vi "仁莫密封检测系统.vi"() -> ()   [LabVIEW 2020]
uses:
  <vilib>/event_ctls.llb/eventvkey.ctl
  <vilib>/NI/Modbus Library/API/Master/Modbus Master.lvclass
  <vilib>/Utility/file.llb/Read Delimited Spreadsheet (string).vi
  <vilib>/NI/Modbus Library/Transmission Data Unit/RTU/RTU Data Unit.lvclass
  <vilib>/NI/Modbus Library/Master Function Definition/Master Function Definition.lvclass
  <vilib>/NI/Modbus Library/Network Protocol/Network Master/Serial/Serial Master.lvclass
panel:
  in  "sn":string
  out "MES状态":bool
  out "通讯状态":bool
  out "泄漏流量":string
  out "参数组别":string
  out "测试时间":string
  out "实时压力":string
  out "泄露压力":string
  out "门限压力":string
  out "目标压力":string
  out "测试 NG":string
  out "测试 OK":string
  out "测试结果":string
  out "测试总量":string
  out "实时压力(图)":dbl(graph)
  out "消息框+":string
  in  "清除计数":bool
  in  "设备启动":bool
  out "运行状态":string
  in  "设备停止":bool
  in  "阻断通讯":bool=TRUE
  out "运行状态":string
  out "失败原因":string
  in  "Exit":bool
  # "仁 莫 密 封 检 测 系 统"
  # "smcc"
  # "S"
  # "Pa"
  # "Pa"
  # "Pa"
  # "Pa"
  # "pcs"
  # "pcs"
  # "pcs"
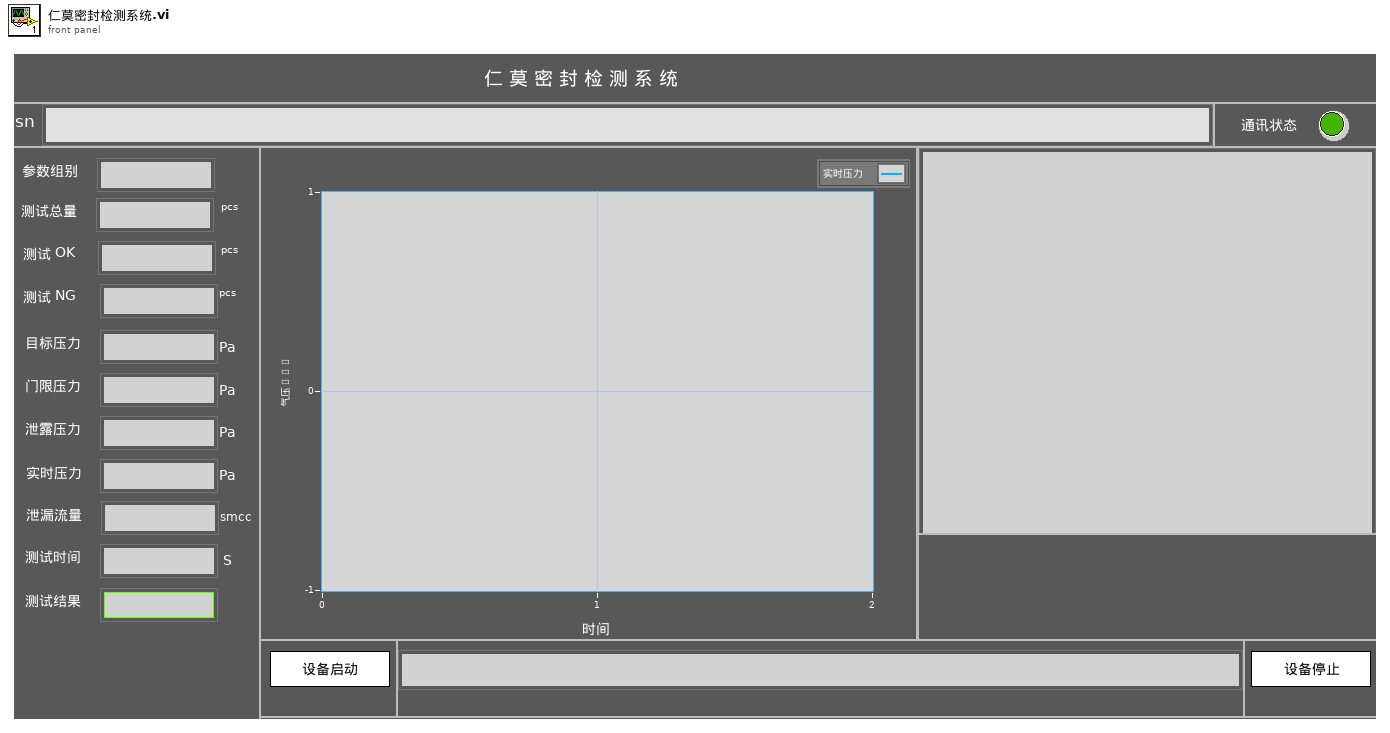
[diagram p1: front panel]
types:
  T1 = typedef "eventvkey.ctl" = enum16{"ASCII", "Enter", "Return", "Shift", "Ctrl", "Alt", "Cmd", "Opt", "Caps", "NumLock", "Clear", "Break", "Up", "Down", "Left", "Right", "Insert", "Delete", "Home", "End", "PageUp", "PageDown", "Escape", "Help", "Pause", "ScrollLock", "F1", "F2", "F3", "F4", "F5", "F6", "F7", "F8", "F9", "F10", "F11", "F12", "F13", "F14", "F15", "F16", "F17", "F18", "F19", "F20", "F21", "F22", "F23", "F24", "Play", "VolumeUp", "VolumeDown", "Mute", "Two Byte Char"}
  T2 = cluster{"地址":u16, "数量":u16, "寄存器值":u16[], "产品总数":string}[]
  T3 = enum32{"Invalid", "Standard", "Closed", "Hidden", "Minimized", "Maximized"}
  T4 = enum32{"invalid app kind", "Development System", "Run Time System", "Student Edition", "Embedded LabVIEW", "Evaluation", "Custom"}
  T5 = cluster{"地址":u16, "数量":u16, "寄存器值":u16[], "名称":string}[]
  T6 = cluster{"读取信息簇":cluster{"地址":u16, "数量":u16, "寄存器值":u16[], "名称":string}, "值解析":string}[]
  T7 = cluster{"温度instance":refnum<class "Modbus Master.lvclass">, "Core":cluster{"Current VI Reference":refnum<vi>, "Close Panel on Exit?":bool}, "serial master instance":refnum<class "Modbus Master.lvclass">, "进站OK":bool, "连接成功":bool, "正在运行":bool, "用户登录":bool, "A读保持寄存器信息组":cluster{"地址":u16, "数量":u16, "寄存器值":u16[], "名称":string}[], "A写入线圈信息组":cluster{"地址":u16, "布尔":bool, "名称":string}[], "A读多组线圈信息组":cluster{"地址":u16, "数量":u16, "名称":string, "线圈组":bool[]}[]}
  T8 = cluster{"连接成功":bool, "MB_实体":refnum<class "Modbus Master.lvclass">}
  T9 = cluster{"地址":u16, "数量":u16, "名称":string, "线圈组":bool[]}[]
  T10 = cluster{"Current VI Reference":refnum<vi>, "Close Panel on Exit?":bool}
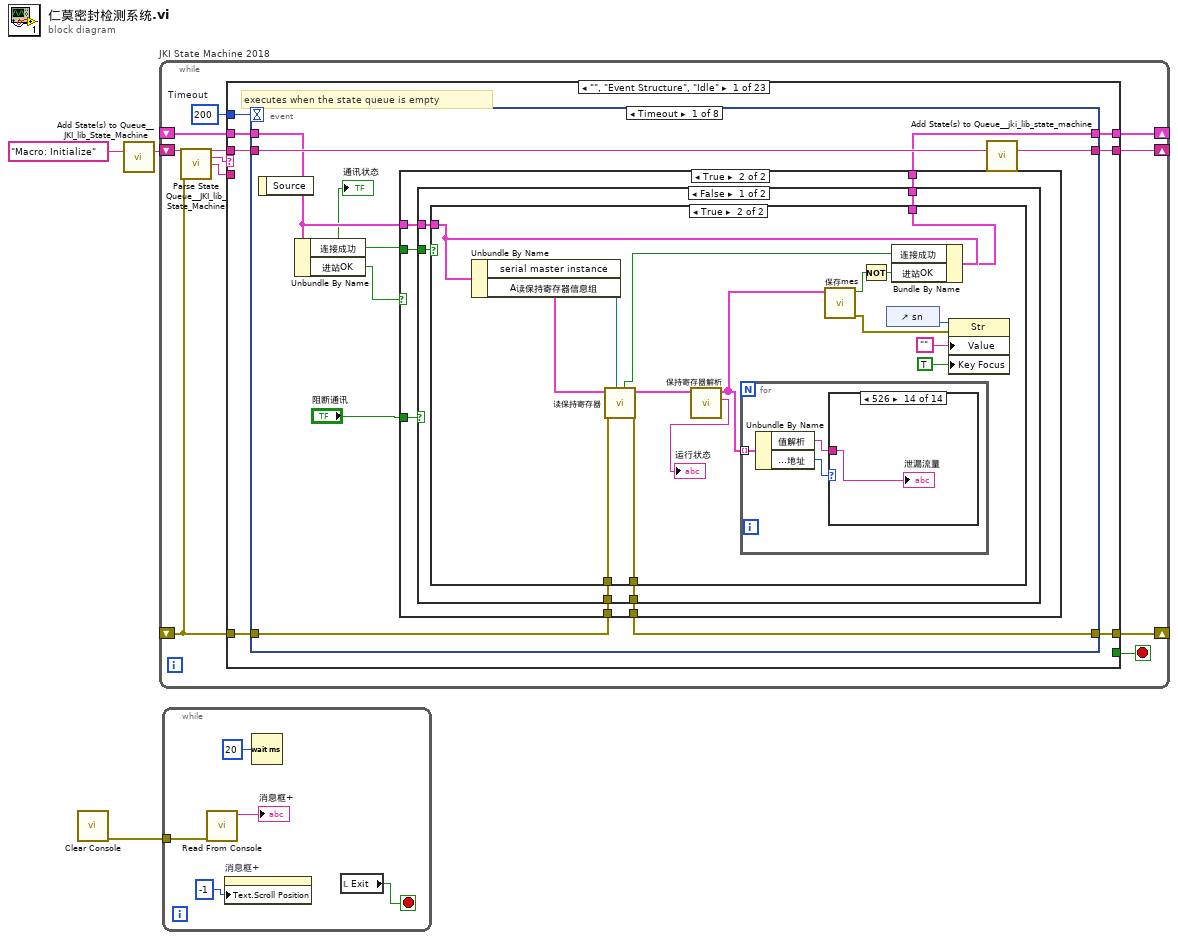
[diagram p0: block diagram]
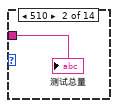
[diagram p5: hidden frame]
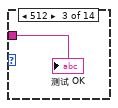
[diagram p6: hidden frame]
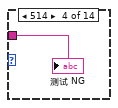
[diagram p7: hidden frame]
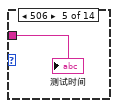
[diagram p8: hidden frame]
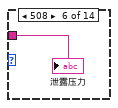
[diagram p9: hidden frame]
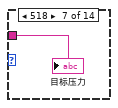
[diagram p10: hidden frame]
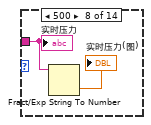
[diagram p11: hidden frame]
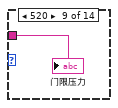
[diagram p12: hidden frame]
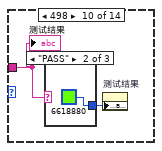
[diagram p13: hidden frame]
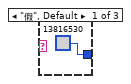
[diagram p14: hidden frame]
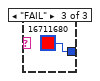
[diagram p15: hidden frame]
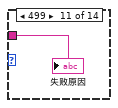
[diagram p16: hidden frame]
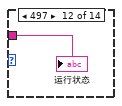
[diagram p17: hidden frame]
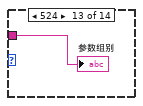
[diagram p18: hidden frame]
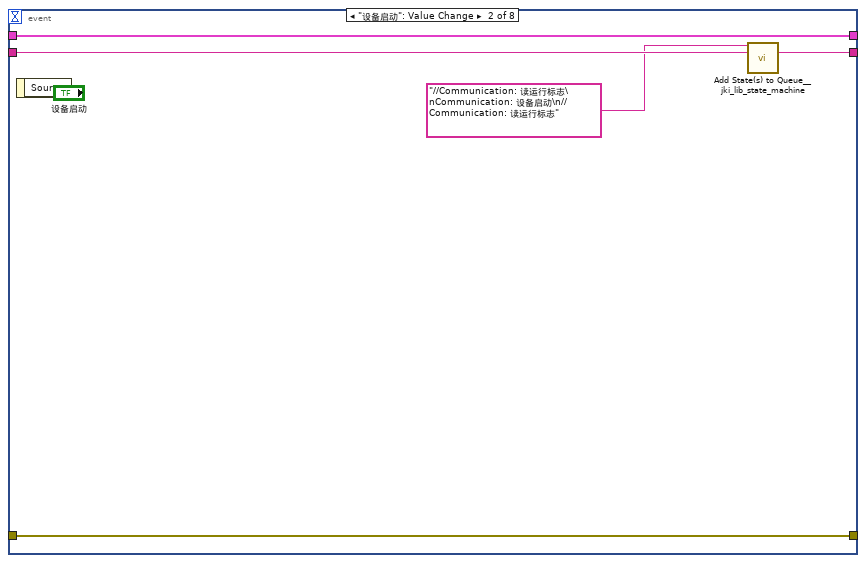
[diagram p20: hidden frame]
diagram:
  n1 = call "Clear Console.vi"() -> ("error out"=w1:errorcluster)  [unwired: 11 in]
  n2 = call <vilib>:"Add State(s) to Queue__JKI_lib_State_Machine.vi"("State(s) in (\"\")"="Macro: Initialize") -> ("States Out"=w3:string)  [unwired: 14 in]
  n3 = while "JKI State Machine 2018" {
    shift-right: [w7] -> _
    shift-left: _ -> [w6]
    shift-right: [w10] -> _
    shift-left: _ -> [w4]
    shift-right: [w9] -> _
    shift-left: w3 -> [w11]
    stop <- w8 stop-if-true
    w5 = 200  # Timeout
    n4 = call <vilib>:"Parse State Queue__JKI_lib_State_Machine.vi"("State Queue"=w11, "Error In (no error)"=w4) -> ("Remaining States"=w13:string, "Current State"=w14:string, "Arguments"=w12:string)  [unwired: 11 in]
    n5 = case shown="\"\", \"Event Structure\", \"Idle\"" w14 {
      selector: w14 -> [_ _ w190 _ _ _ _ _ _ _ _ _ _ _ _ _ _ _ _ _ _ _ _]
      tunnel: w13 -> [w21 w189 w194 w213 w220 w225 w229 w250 w259 w263 w277 w283 w294 w363 w368 w378 w382 w394 w406 w453 w485 w497 w502]
      tunnel: w12 -> [_ _ _ _ _ _ _ _ _ _ _ w278 w288 _ _ _ _ _ _ _ _ _ _]
      tunnel: w6 -> [w19 w186 w192 w206 w217 w223 w226 _ w255 w260 w275 w281 w290 w360 w365 w375 w379 w388 w400 w447 w478 w494 w499]
      tunnel: [w18 w187 w196 w210 errorcluster {"status"=FALSE, "code"=0, "source"=""} ("error out") w222 w227 w247 w256 w261 w274 w279 w291 w361 w366 w376 w380 w383 w403 w450 w482 w495 w500] -> w10
      tunnel: w4 -> [w17 w187 w195 w210 w215 w222 w227 w247 w253 w261 w274 w280 w292 w361 w366 w376 w380 w391 w404 w451 w483 w495 w500]
      tunnel: [w20 w188 w193 w212 w219 w224 w228 w249 w258 w262 w276 w282 w293 w362 w367 w377 w381 w393 w405 w452 w484 w496 w501] -> w9
      tunnel: [_ _ _ _ _ w221 _ _ _ _ _ _ _ _ _ _ _ _ _ _ _ _ _] -> w8
      tunnel: [w16 w186 w192 w211 w217 w223 w226 w248 w255 w260 w275 w281 w290 w360 w365 w375 w379 w386 w398 w445 w479 w494 w498] -> w7
      tunnel: w5 -> [w15 _ _ _ _ _ _ _ _ _ _ _ _ _ _ _ _ _ _ _ _ _ _]
      frame "", "Event Structure", "Idle" {
        # "executes when the state queue is empty"
        n6 = event shown="[0] Timeout" {
          selector: _ -> [_ _ _ _ _ _ _ _]
          dyn-events: _ -> [_ _ _ _ _ _ _ _]
          timeout: w15 -> [_ _ _ _ _ _ _ _]
          tunnel: w21 -> [w30 w89 w94 w100 w155 w169 w179 w185]
          tunnel: [w29 w88 w93 w99 w154 w168 w178 w184] -> w20
          tunnel: w19 -> [w28 w86 w91 w96 w152 w164 w176 w182]
          tunnel: [w26 w87 w92 w98 w153 w161 w177 w183] -> w18
          tunnel: w17 -> [w27 w87 w92 w98 w153 w162 w177 w183]
          tunnel: [w25 w86 w91 w95 w151 w163 w176 w182] -> w16
          event Timeout {
            n7 = event-data() -> ()  [unwired: 1 in, 1 out]
            n8 = Unbundle By Name(w28) -> ("连接成功"=w23:bool, "进站OK"=w22:bool)
            "通讯状态" <- w23
            n9 = case shown="True" w22 {
              tunnel: w28 -> [w32 w38]
              tunnel: w27 -> [w31 w37]
              tunnel: [w31 w36] -> w26
              tunnel: [w32 w35] -> w25
              tunnel: "阻断通讯" -> [_ w34]
              tunnel: w23 -> [_ w33]
              frame False {
              }
              frame True {
                n10 = case shown="False" w34 {
                  tunnel: w33 -> [w43 _]
                  tunnel: w38 -> [w42 w83]
                  tunnel: w37 -> [w41 w84]
                  tunnel: [w40 w84] -> w36
                  tunnel: [w39 w83] -> w35
                  frame False {
                    n11 = case shown="True" w43 {
                      tunnel: w42 -> [w44 w59]
                      tunnel: w41 -> [w45 w61]
                      tunnel: [w45 w60] -> w40
                      tunnel: [w44 w54] -> w39
                      frame False {
                      }
                      frame True {
                        n12 = Unbundle By Name(w59) -> ("serial master instance"=w58:refnum<class "Modbus Master.lvclass">, "A读保持寄存器信息组"=w57:T5)
                        n13 = call "读保持寄存器.vi"("MB_实体"=w58, "error in"=w61, "读保持寄存器信息组__输入"=w57) -> ("输出簇"=w60:errorcluster, "读保持寄存器信息组_输出"=w55:T5, "连接成功"=w56:bool)  [unwired: 6 in]
                        n14 = call "保持寄存器解析.vi"("A读保持寄存器信息组"=w55) -> ("运行状态"=→"运行状态":string, "参数值"=w53:T6)  [unwired: 9 in]
                        n15 = for {
                          tunnel: w53 -> [w63] mode=indexing
                          n16 = Unbundle By Name(w63) -> ("值解析"=w62:string, "读取信息簇.地址"=w64:u16)
                          n17 = case shown="526" w64 {
                            tunnel: w62 -> [_ w65 w66 w67 w68 w69 w70 w72 w73 w75 w79 w80 w81 w82]
                            frame Default {
                            }
                            frame 510 {
                              "测试总量" <- w65
                            }
                            frame 512 {
                              "测试 OK" <- w66
                            }
                            frame 514 {
                              "测试 NG" <- w67
                            }
                            frame 506 {
                              "测试时间" <- w68
                            }
                            frame 508 {
                              "泄露压力" <- w69
                            }
                            frame 518 {
                              "目标压力" <- w70
                            }
                            frame 500 {
                              n18 = Fract/Exp String To Number(string=w72) -> (number=→"实时压力(图)":dbl)  [unwired: 3 in, 1 out]
                              "实时压力" <- w72
                            }
                            frame 520 {
                              "门限压力" <- w73
                            }
                            frame 498 {
                              n19 = case shown="\"PASS\"" w75 {
                                tunnel: [u32 13816530 ("颜色盒") u32 6618880 u32 16711680] -> w74
                                frame "假", Default {
                                }
                                frame "PASS" {
                                }
                                frame "FAIL" {
                                }
                              }
                              n20 = property on="测试结果" class="Str"("Text.BGColor"=w74) -> ()  [unwired: 2 in, 2 out]
                              "测试结果" <- w75
                            }
                            frame 499 {
                              "失败原因" <- w79
                            }
                            frame 497 {
                              "运行状态" <- w80
                            }
                            frame 524 {
                              "参数组别" <- w81
                            }
                            frame 526 {
                              "泄漏流量" <- w82
                            }
                          }
                        }
                        n21 = call "保存mes.vi"("参数值"=w53) -> ("error out"=w48:errorcluster, "出站成功"=w51:bool)  [unwired: 9 in]
                        n22 = Not(x=w51) -> (.not. x?=w50:bool)
                        n23 = control-ref of="sn"() -> (w49:refnum<vi>)
                        n24 = Bundle By Name(cluster=w59, "连接成功"=w56, "进站OK"=w50) -> (w54:T7)
                        n25 = property on="属性节点" class="Str"(reference=w49, error in=w48, "Value"="", "Key Focus"=TRUE ("键选中")) -> ()  [unwired: 2 out]
                      }
                    }
                  }
                  frame True {
                  }
                }
              }
            }
            n26 = call <vilib>:"Add State(s) to Queue__jki_lib_state_machine.vi"("State(s) in (\"\")"=w30) -> ("States Out"=w29:string)  [unwired: 14 in]
          }
          event "设备启动": Value Change {
            n27 = event-data() -> ()  [unwired: 1 in, 1 out]
            n28 = call <vilib>:"Add State(s) to Queue__jki_lib_state_machine.vi"("State(s) in Front (\"\")"="//Communication: 读运行标志\nCommunication: 设备启动\n//Communication: 读运行标志", "State(s) in (\"\")"=w89) -> ("States Out"=w88:string)  [unwired: 13 in]
          }
          event "设备停止": Value Change {
            n29 = event-data() -> ()  [unwired: 1 in, 1 out]
            n30 = call <vilib>:"Add State(s) to Queue__jki_lib_state_machine.vi"("State(s) in Front (\"\")"="//Communication: 读运行标志\nCommunication: 设备停止\n//Communication: 读运行标志", "State(s) in (\"\")"=w94) -> ("States Out"=w93:string)  [unwired: 13 in]
          }
          event Menu Selection (User) {
            n31 = event-data() -> ("ItemTag"=w97:string)  [unwired: 1 in]
            n32 = case shown="\"历史数据路径配置\"" w97 {
              tunnel: w96 -> [w101 w102 w113 w124 w125 w127 w138]
              tunnel: [w101 w102 w113 w124 w125 w126 w137] -> w95
              frame "假", Default {
              }
              frame "历史数据查询" {
                n33 = stacked-sequence {
                  frame #0 {
                    n34 = call <vilib>:"Check if File or Folder Exists.vi"("path"=path "D:/MES" ("路径")) -> ("file or folder exists?"=w105:bool, "dup path"=w104:path)  [unwired: 8 in, 1 out]
                    n35 = case shown="False" w105 {
                      tunnel: w104 -> [w107 w108]
                      tunnel: [w106 w108] -> _
                      frame False {
                        n36 = Create Folder(path (use dialog)=w107) -> (created path=w106:path)  [unwired: 2 in, 2 out]
                      }
                      frame True {
                      }
                    }
                  }
                  frame #1 {
                    n37 = call <vilib>:"Space Constant.vi"() -> ("String"=w110:string)
                    n38 = Concatenate Strings("explorer" ("字符串"), w110, "D:\\MES" ("字符串")) -> (w112:string)
                    n39 = call <vilib>:"System Exec.vi"("command line"=w112) -> ()  [unwired: 7 in, 4 out]
                  }
                }
              }
              frame "MES日志查询" {
                n40 = stacked-sequence {
                  frame #0 {
                    n41 = call <vilib>:"Check if File or Folder Exists.vi"("path"=path "D:/Log" ("路径")) -> ("file or folder exists?"=w116:bool, "dup path"=w115:path)  [unwired: 8 in, 1 out]
                    n42 = case shown="False" w116 {
                      tunnel: w115 -> [w118 w119]
                      tunnel: [w117 w119] -> _
                      frame False {
                        n43 = Create Folder(path (use dialog)=w118) -> (created path=w117:path)  [unwired: 2 in, 2 out]
                      }
                      frame True {
                      }
                    }
                  }
                  frame #1 {
                    n44 = call <vilib>:"Space Constant.vi"() -> ("String"=w121:string)
                    n45 = Concatenate Strings("explorer" ("字符串"), w121, "D:\\Log" ("字符串")) -> (w123:string)
                    n46 = call <vilib>:"System Exec.vi"("command line"=w123) -> ()  [unwired: 7 in, 4 out]
                  }
                }
              }
              frame "IP配置" {
                n47 = call "IP配置.vi"() -> ()  [unwired: 11 in, 1 out]
              }
              frame "历史数据路径配置" {
                n48 = call "Path配置.vi"() -> ()  [unwired: 11 in, 1 out]
              }
              frame "通讯参数设置" {
                n49 = stacked-sequence {
                  tunnel: w127 -> [_ w132 _]
                  tunnel: [_ w129 _] -> w126
                  frame #0 {
                    n50 = local write "阻断通讯"(TRUE ("阻断通讯")) -> ()
                  }
                  frame #1 {
                    n51 = call "通讯参数设置.vi"() -> ("A设备簇"=w133:T8)  [unwired: 5 in]
                    n52 = Unbundle By Name(w133) -> ("MB_实体"=w131:refnum<class "Modbus Master.lvclass">, "连接成功"=w130:bool)
                    n53 = Bundle By Name(cluster=w132, "serial master instance"=w131, "连接成功"=w130) -> (w129:T7)
                  }
                  frame #2 {
                    n54 = local write "阻断通讯"(FALSE ("阻断通讯")) -> ()
                  }
                }
              }
              frame "本地控制" {
                n55 = call "本地控制.vi"() -> ("远程2"=w136:bool)  [unwired: 11 in]
                "MES状态" <- w136
                n56 = Not(x=w136) -> (.not. x?=w135:bool)
                n57 = Bundle By Name(cluster=w138, "用户登录"=w135, "进站OK"=w135) -> (w137:T7)
                n58 = global write "Global.vi" "产品进站"(w135) -> ()
                n59 = case shown="True" w136 {
                  frame False {
                    n60 = Current VI's Menubar() -> (w140:refnum<k9>)
                    n61 = Delete Menu Items(9:w140) -> (3:w139:refnum<k9>)  [unwired: 3 in, 1 out]
                    n62 = Insert Menu Items(7:string[] ["历史数据查询", "通讯参数设置", "MES配置", "MES日志查询", "本地控制", "温湿度设置"] ("L10n_item tags 1"), 9:w139) -> ()  [unwired: 4 in, 3 out]
                  }
                  frame True {
                    n63 = Current VI's Menubar() -> (w144:refnum<k9>)
                    n64 = Delete Menu Items(9:w144) -> (0:w142:errorcluster, 3:w143:refnum<k9>)  [unwired: 3 in]
                    n65 = Insert Menu Items(6:w142, 7:string[] ["用户登录", "历史数据查询", "通讯参数设置", "MES配置", "MES日志查询", "本地控制", "温湿度设置"] ("L10n_item tags 1"), 9:w143) -> ()  [unwired: 3 in, 3 out]
                  }
                }
              }
            }
            n66 = call <vilib>:"Add State(s) to Queue__jki_lib_state_machine.vi"("State(s) in (\"\")"=w100) -> ("States Out"=w99:string)  [unwired: 14 in]
          }
          event "sn": Key Down {
            n67 = event-data() -> ("VKey"=w150:T1)  [unwired: 1 in]
            n68 = Equal?(x=w150, y=eventvkey."Return" ("V键")) -> (x = y?=w148:bool)
            n69 = case shown="True" w148 {
              tunnel: [FALSE ("进站成功") TRUE ("进站成功")] -> w147
              frame False {
              }
              frame True {
                n70 = global write "Global.vi" "sn"("sn") -> ()
              }
            }
            n71 = global write "Global.vi" "产品进站"(w147) -> ()
            n72 = Bundle By Name(cluster=w152, "进站OK"=w147) -> (w151:T7)
            n73 = case shown="True" w147 {
              tunnel: ["" "Communication: 设备启动"] -> w146
              frame False {
              }
              frame True {
              }
            }
            n74 = call <vilib>:"Add State(s) to Queue__jki_lib_state_machine.vi"("State(s) in (\"\")"=w155, "State(s) at Back (\"\")"=w146) -> ("States Out"=w154:string)  [unwired: 13 in]
          }
          event "清除计数": Value Change {
            n75 = event-data() -> ()  [unwired: 1 in, 1 out]
            n76 = local write "清除计数"(FALSE) -> ()
            n77 = Unbundle By Name(w164) -> ("serial master instance"=w165:refnum<class "Modbus Master.lvclass">)
            n78 = disable-structure shown="禁用" {
              disable-tunnel: [w174 _] -> w166
              disable-tunnel: w165 -> [w173 _]
              disable-tunnel: w162 -> [w171 _]
              disable-tunnel: [w170 _] -> w161
              frame Disabled {
                n79 = call "写保持寄存器.vi"("MB_实体"=w173, "error in"=w171, "读保持寄存器信息组__输入"=T2 [{"地址"=510, "数量"=2, "寄存器值"=[0, 0], "产品总数"="产品总数"}, {"地址"=512, "数量"=2, "寄存器值"=[0, 0], "产品总数"="合格数量"}, {"地址"=514, "数量"=2, "寄存器值"=[0, 0], "产品总数"="泄露数量"}]) -> ("输出簇"=w170:errorcluster, "连接成功"=w174:bool)  [unwired: 7 in]
              }
              frame Enabled {
              }
            }
            n80 = Bundle By Name(cluster=w164, "连接成功"=w166) -> (w163:T7)
            n81 = call <vilib>:"Add State(s) to Queue__jki_lib_state_machine.vi"("State(s) in (\"\")"=w169) -> ("States Out"=w168:string)  [unwired: 14 in]
          }
          event "Exit": Value Change {
            # "Exit Button Value Change (pressed) Event\n(this executes Macro: Exit to terminate the VI)"
            n82 = event-data() -> ()  [unwired: 1 in, 1 out]
            n83 = call <vilib>:"Add State(s) to Queue__jki_lib_state_machine.vi"("State(s) in Front (\"\")"="Macro: Exit", "State(s) in (\"\")"=w179) -> ("States Out"=w178:string)  [unwired: 13 in]
          }
          event Panel Close? {
            # "Discard the event because we'll close the front panel ourselves in Macro: Exit"
            # "Close Panel button (pressed) Event\n(this executes Macro: Exit to terminate the VI)"
            n84 = event-data() -> ()  [unwired: 1 in, 1 out]
            n85 = call <vilib>:"Add State(s) to Queue__jki_lib_state_machine.vi"("State(s) in Front (\"\")"="Macro: Exit", "State(s) in (\"\")"=w185) -> ("States Out"=w184:string)  [unwired: 13 in]
            n86 = event-data("Discard?"=TRUE) -> ()  [unwired: 1 in, 1 out]
          }
        }
      }
      frame "---------- Core ----------" {
        # "Do not put any code in this frame.\n(it is a separator no-op)"
        n87 = call <vilib>:"Add State(s) to Queue__jki_lib_state_machine.vi"("State(s) in (\"\")"=w189) -> ("States Out"=w188:string)  [unwired: 14 in]
      }
      frame Default {
        w199 = 42 items=["No error", "Argument error", "Memory is full", "Out of zone", "End of file", "File already open", "Generic file I/O error", "File not found", "File permission error", "Disk is full", "Duplicate path", "Too many files open", "System feature not enabled", "Resource file not found", "Cannot add resource", "Resource not found", "Image not found", "Image memory error", "Pen does not exist", "Config type invalid", "Config token not found", "Config parse error", "Config memory error", "Bad external code format", "Bad external code offset", "External code not present", "Null window", "Destroy window error", "Null menu", "Print aborted", "Bad print record", "Print driver error", "Windows error during printing", "Memory error during printing", "Print dialog error", "Generic print error", "Invalid device refnum", "Device not found", "Device parameter error", "Device unit error", "Cannot open device", "Device call aborted", "Generic error", "Cancelled by user", "Object ID too low", "Object ID too high", "Object not in heap", "Unknown heap", "Unknown object (invalid DefProc)", "Unknown object (DefProc not in table)", "Message out of range", "Invalid (null) method", "Unknown message", "Manager call not supported", "Bad address", "Network operation in progress", "Network operation timed out", "Connection is busy", "Network attribute not supported", "Network error", "Address in use", "System out of memory", "Connection aborted", "Connection refused", "Not connected", "Already connected", "Connection closed", "Initialization error (interapplication manager)", "Bad occurrence", "Wait on unbound occurrence handler", "Occurrence queue overflow", "Datalog type conflict", "Unused", "Unrecognized type (interapplication manager)", "Memory corrupt", "Failed to make temporary DLL", "Old CIN version", "Drag socket not found", "Failed to load drop-object", "Failed to register OLE object", "Failed to release OLE object", "Format specifier type mismatch", "Unknown format specifier", "Too few format specifiers", "Too many format specifiers", "Scan failed", "Newer CIN version", "Error converting to variant", "Runtime menu error", "Password tampered", "Variant attribute not found", "Incompatible variant data type", "Event data is not available", "Event Store is not present", "Occurrence is not found", "Event Queue is not created", "Event info is not available", "Refnum passed is NULL", "Error retrieving Class GUID", "Error retrieving CoClass GUID", "Error retrieving TypeLib GUID.", "Bad built application magic bytes.", "Specific driver is different from the specific driver associated with the Logical Name.", "There is no session opened to the class driver.", "Max Error", "MAX - Error with config objects", "MAX - Error loading configuration", "MAX - Group not supported"]
        # "Current State"
        # "Do not delete, rename, or modify this frame.\n(this is used to capture unhandled states and typos)"
        # "Handle mistyped state name (developer tool)"
        n88 = Format Into String(format string="Software Exception: Unhandled State \"%s\"." ("message"), error in=w195, w190) -> (resulting string=w198:string, error out=w197:errorcluster)  [unwired: 1 in]
        n89 = call <vilib>:"Error Cluster From Error Code.vi"("show call chain? (False)"=TRUE, "error in (no error)"=w197, "error message (\"\")"=w198, "error code (0)"=w199) -> ("error out"=w196:errorcluster)  [unwired: 5 in]
        n90 = call <vilib>:"Add State(s) to Queue__jki_lib_state_machine.vi"("State(s) in (\"\")"=w194) -> ("States Out"=w193:string)  [unwired: 14 in]
      }
      frame "Initialize Core Data" {
        # "Do not delete, rename, or modify this frame.\n(this is used to determine panel behavior on exit)"
        # "originally closed?"
        # "exe?"
        # "If panel starts closed or is an EXE, then close it when we exit"
        n91 = property class="VI"() -> ("FP.State"=w203:T3)  [unwired: 2 in, 2 out]
        n92 = property class="App"() -> ("App.Kind"=w209:T4)  [unwired: 2 in, 2 out]
        n93 = control-ref of="Current VI Reference"() -> (w204:refnum<vi>)
        n94 = Equal?(x=w203, y=T3."Closed" ("Front Panel Window:State")) -> (x = y?=w201:bool)
        n95 = Equal?(x=w209, y=T4."Run Time System" ("Application:Kind")) -> (x = y?=w207:bool)
        n96 = Or(x=w201, y=w207) -> (x .or. y?=w205:bool)
        n97 = Bundle By Name(cluster=w206, "Core.Current VI Reference"=w204, "Core.Close Panel on Exit?"=w205) -> (w211:T7)
        n98 = call <vilib>:"Add State(s) to Queue__jki_lib_state_machine.vi"("State(s) in (\"\")"=w213) -> ("States Out"=w212:string)  [unwired: 14 in]
      }
      frame "Error Handler" {
        # "Handle any errors here.\nYou can also output any states to clean-up after errors occur"
        # "Clear error"
        n99 = Unbundle By Name(w215) -> ("source"=w214:string)
        n100 = One Button Dialog(message=w214) -> ()  [unwired: 1 in, 1 out]
        n101 = call <vilib>:"Add State(s) to Queue__jki_lib_state_machine.vi"("State(s) in Front (\"\")"="/* Post Error States", "State(s) in (\"\")"=w220) -> ("States Out"=w219:string)  [unwired: 13 in]
      }
      frame "Exit" {
        w221 = TRUE
        # "Do not put any code in this frame.\n(No errors that occur here will be handled.)"
        n102 = local write "Exit"(w221) -> ()
        n103 = call <vilib>:"Add State(s) to Queue__jki_lib_state_machine.vi"("State(s) in (\"\")"=w225) -> ("States Out"=w224:string)  [unwired: 14 in]
      }
      frame "---------- Data ----------" {
        # "Do not put any code in this frame.\n(It is a separator no-op. You can make a copy of this frame to create a new Data frame)"
        n104 = call <vilib>:"Add State(s) to Queue__jki_lib_state_machine.vi"("State(s) in (\"\")"=w229) -> ("States Out"=w228:string)  [unwired: 14 in]
      }
      frame "Data: Initialize" {
        w230 = refnum<class "Modbus Master.lvclass"> refnum  # 温度instance
        w231 = FALSE ("MES状态")
        w232 = FALSE  # 进站OK
        w239 = TRUE  # 用户登录
        w240 = FALSE  # 正在运行
        w241 = T5 [{"地址"=510, "数量"=2, "寄存器值"=[0, 0], "名称"="产品总数"}, {"地址"=512, "数量"=2, "寄存器值"=[0, 0], "名称"="合格数量"}, {"地址"=514, "数量"=2, "寄存器值"=[0, 0], "名称"="泄露数量"}, {"地址"=506, "数量"=2, "寄存器值"=[0, 0], "名称"="1测试时间"}, {"地址"=508, "数量"=2, "寄存器值"=[0, 0], "名称"="1测试泄漏"}, {"地址"=518, "数量"=2, "寄存器值"=[0, 0], "名称"="1#目标压力"}, {"地址"=498, "数量"=1, "寄存器值"=[0, 0], "名称"="1#测试结果"}, {"地址"=500, "数量"=2, "寄存器值"=[0, 0], "名称"="实时压力"}, {"地址"=520, "数量"=2, "寄存器值"=[], "名称"="门限压力"}, {"地址"=499, "数量"=1, "寄存器值"=[], "名称"="失败原因"}, {"地址"=497, "数量"=1, "寄存器值"=[], "名称"="运行状态"}, {"地址"=524, "数量"=2, "寄存器值"=[], "名称"="参数组别"}, {"地址"=526, "数量"=4, "寄存器值"=[], "名称"="泄漏流量"}]  # A读保持寄存器信息组
        w242 = T9 [{"地址"=507, "数量"=1, "名称"="1测试结束标志", "线圈组"=[FALSE, TRUE]}]  # A读多组线圈信息组
        w243 = cluster{"地址":u16, "布尔":bool, "名称":string}[] [{"地址"=50, "布尔"=FALSE, "名称"="启动"}, {"地址"=51, "布尔"=FALSE, "名称"="停止"}]  # A写入线圈信息组
        w244 = FALSE  # 连接成功
        w245 = refnum<class "Modbus Master.lvclass"> refnum  # serial master instance
        w246 = T10 {"Current VI Reference"=refnum, "Close Panel on Exit?"=FALSE}  # Core
        # "Initialize the shift-register data, here.\n(data names are defined by what you wire into the bundle function)"
        n105 = call <vilib>:"Application Directory.vi"() -> ("Application Directory"=w237:path)
        n106 = Build Path(base path=w237, name or relative path=path "data/mes.cfg") -> (appended path=w238:path)
        n107 = call-poly <vilib>:"Read Delimited Spreadsheet.vi"("file path (dialog if empty)"=w238, "delimiter (\\t)"="::" ("delimiter (\\t)")) -> ("all rows"=w233:string[][])  [unwired: 8 in, 5 out]
        n108 = call "mes初始化.vi"("mes"=w233) -> ()  [unwired: 11 in]
        n109 = disable-structure shown="禁用" {
          frame Disabled {
            n110 = global write "Global.vi" "MES状态"(TRUE ("MES状态")) -> ()
          }
          frame Enabled {
          }
        }
        n111 = global write "Global.vi" "正在运行"(w231) -> ()
        n112 = global write "Global.vi" "产品进站"(w231) -> ()
        n113 = global write "Global.vi" "运行状态时间点"(dbl[] [0.0, 0.0, 0.0, 0.0, 0.0, 0.0, 0.0, 0.0, 0.0] ("运行状态时间点")) -> ()
        n114 = Bundle("温度instance"=w230, "Core"=w246, "serial master instance"=w245, "进站OK"=w232, "连接成功"=w244, "正在运行"=w240, "用户登录"=w239, "A读保持寄存器信息组"=w241, "A写入线圈信息组"=w243, "A读多组线圈信息组"=w242) -> (w248:T7)  [unwired: 1 in]
        n115 = call <vilib>:"Add State(s) to Queue__jki_lib_state_machine.vi"("State(s) in (\"\")"=w250) -> ("States Out"=w249:string)  [unwired: 14 in]
      }
      frame "Data: Cleanup" {
        # "Cleanup any data and references, here.\n(this is called automatically, by the Macro: Exit)"
        n116 = Unbundle By Name(w255) -> ("Core.Current VI Reference"=w257:refnum<vi>, "serial master instance"=w254:refnum<class "Modbus Master.lvclass">)
        n117 = call-dynamic "Shutdown.vi"("error in"=w253, "Modbus master in"=w254) -> ("error out"=w252:errorcluster)  [unwired: 9 in]
        n118 = Close Reference(reference=w257, error in (no error)=w252) -> (error out=w256:errorcluster)
        n119 = call <vilib>:"Add State(s) to Queue__jki_lib_state_machine.vi"("State(s) in (\"\")"=w259) -> ("States Out"=w258:string)  [unwired: 14 in]
      }
      frame "---------- UI ----------" {
        # "Do not put any code in this frame.\n(It is a separator no-op. You can make a copy of this frame to create a new UI frame)"
        n120 = call <vilib>:"Add State(s) to Queue__jki_lib_state_machine.vi"("State(s) in (\"\")"=w263) -> ("States Out"=w262:string)  [unwired: 14 in]
      }
      frame "UI: Initialize" {
        # "Initialize the User Interface, here.\n(this is called automatically, by the Macro: Init)"
        n121 = call "读取配置文件.vi"("配置"="程序名") -> ("error out"=w270:errorcluster, "路径"=w269:string)  [unwired: 9 in]
        n122 = property class="VI"(error in=w270, "Front Panel.Title"=w269) -> (error out=w267:errorcluster)  [unwired: 1 in, 1 out]
        n123 = Current VI's Menubar() -> (w273:refnum<k9>)
        n124 = Delete Menu Items(6:w267, 9:w273) -> (0:w272:errorcluster, 3:w271:refnum<k9>)  [unwired: 2 in]
        n125 = local write "sn"("") -> ()
        n126 = Insert Menu Items(6:w272, 7:string[] ["通讯参数设置", "IP配置", "历史数据路径配置"] ("L10n_item tags 1"), 9:w271) -> ()  [unwired: 3 in, 3 out]
        n127 = property on="测试结果" class="Str"("Text.BGColor"=u32 13816530 ("颜色盒")) -> ()  [unwired: 2 in, 2 out]
        n128 = call <vilib>:"Add State(s) to Queue__jki_lib_state_machine.vi"("State(s) in (\"\")"=w277) -> ("States Out"=w276:string)  [unwired: 14 in]
      }
      frame "UI: Cursor Set" {
        # "Argument"
        # "Set and Unset Cursor Busy.\n(Usage: \"UI: Cursor Set >> Busy|Idle\")"
        n129 = case shown="\"Idle\", Default" w278 {
          tunnel: w280 -> [w285 w287]
          tunnel: [w284 w286] -> w279
          frame "Idle", Default {
            n130 = call <vilib>:"Unset Busy.vi"("error in (no error)"=w285) -> ("error out"=w284:errorcluster)  [unwired: 10 in]
          }
          frame "Busy" {
            n131 = call <vilib>:"Set Busy.vi"("error in (no error)"=w287) -> ("error out"=w286:errorcluster)  [unwired: 9 in, 1 out]
          }
        }
        n132 = call <vilib>:"Add State(s) to Queue__jki_lib_state_machine.vi"("State(s) in (\"\")"=w283) -> ("States Out"=w282:string)  [unwired: 14 in]
      }
      frame "UI: Front Panel State" {
        # "Argument"
        # "Set Front Panel Open or Closed\n(Usage: \"UI: Front Panel State >> Open|Close\")"
        n133 = Unbundle By Name(w290) -> ("Core.Current VI Reference"=w289:refnum<vi>)
        n134 = case shown="\"Maximize\", \"Maximized\"" w288 {
          tunnel: w292 -> [w300 w315 w326 w339 w352]
          tunnel: [w302 w316 w328 w341 w354] -> w291
          tunnel: w289 -> [w301 w313 w327 w340 w353]
          frame "Open", "Standard", Default {
            w295 = T3."Standard" ("State")
            n135 = property class="VI"(reference=w301, error in=w300) -> (reference out=w298:refnum<vi>, error out=w299:errorcluster, "FP.State"=w297:T3)
            n136 = Not Equal?(x=w297, y=w295) -> (x != y?=w296:bool)
            n137 = case shown="True" w296 {
              tunnel: [w306 w308] -> w302
              tunnel: w299 -> [w305 w308]
              tunnel: w298 -> [w304 _]
              tunnel: w295 -> [w303 _]
              frame True {
                n138 = invoke class="VI" method="FP.Open"(reference=w304, error in=w305, "Activate"=TRUE, "State"=w303) -> (error out=w306:errorcluster)  [unwired: 1 in, 4 out]
              }
              frame False {
              }
            }
          }
          frame "Close", "Closed" {
            n139 = property class="VI"(reference=w313, error in=w315) -> (reference out=w312:refnum<vi>, error out=w314:errorcluster, "FP.State"=w310:T3)
            n140 = Not Equal?(x=w310, y=T3."Closed" ("Front Panel Window:State")) -> (x != y?=w309:bool)
            n141 = case shown="True" w309 {
              tunnel: [w317 w320] -> w316
              tunnel: w314 -> [w317 w319]
              tunnel: w312 -> [_ w318]
              frame False {
              }
              frame True {
                n142 = invoke class="VI" method="FP.Close"(reference=w318, error in=w319) -> (error out=w320:errorcluster)  [unwired: 1 in, 2 out]
              }
            }
          }
          frame "Hidden", "Hide" {
            w321 = T3."Hidden" ("State")
            n143 = property class="VI"(reference=w327, error in=w326) -> (reference out=w324:refnum<vi>, error out=w325:errorcluster, "FP.State"=w323:T3)
            n144 = Not Equal?(x=w323, y=w321) -> (x != y?=w322:bool)
            n145 = case shown="True" w322 {
              tunnel: [w332 w333] -> w328
              tunnel: w325 -> [w331 w333]
              tunnel: w324 -> [w330 _]
              tunnel: w321 -> [w329 _]
              frame True {
                n146 = invoke class="VI" method="FP.Open"(reference=w330, error in=w331, "State"=w329) -> (error out=w332:errorcluster)  [unwired: 2 in, 4 out]
              }
              frame False {
              }
            }
          }
          frame "Minimize", "Minimized" {
            w334 = T3."Minimized" ("State")
            n147 = property class="VI"(reference=w340, error in=w339) -> (reference out=w337:refnum<vi>, error out=w338:errorcluster, "FP.State"=w336:T3)
            n148 = Not Equal?(x=w336, y=w334) -> (x != y?=w335:bool)
            n149 = case shown="True" w335 {
              tunnel: [w345 w346] -> w341
              tunnel: w338 -> [w344 w346]
              tunnel: w337 -> [w343 _]
              tunnel: w334 -> [w342 _]
              frame True {
                n150 = invoke class="VI" method="FP.Open"(reference=w343, error in=w344, "State"=w342) -> (error out=w345:errorcluster)  [unwired: 2 in, 4 out]
              }
              frame False {
              }
            }
          }
          frame "Maximize", "Maximized" {
            w347 = T3."Maximized" ("State")
            n151 = property class="VI"(reference=w353, error in=w352) -> (reference out=w350:refnum<vi>, error out=w351:errorcluster, "FP.State"=w349:T3)
            n152 = Not Equal?(x=w349, y=w347) -> (x != y?=w348:bool)
            n153 = case shown="True" w348 {
              tunnel: [w358 w359] -> w354
              tunnel: w351 -> [w357 w359]
              tunnel: w350 -> [w356 _]
              tunnel: w347 -> [w355 _]
              frame True {
                n154 = invoke class="VI" method="FP.Open"(reference=w356, error in=w357, "State"=w355) -> (error out=w358:errorcluster)  [unwired: 2 in, 4 out]
              }
              frame False {
              }
            }
          }
        }
        n155 = call <vilib>:"Add State(s) to Queue__jki_lib_state_machine.vi"("State(s) in (\"\")"=w294) -> ("States Out"=w293:string)  [unwired: 14 in]
      }
      frame "---------- Macro ----------" {
        # "Do not put any code in this frame.\n(It is a separator no-op. You can make a copy of this frame to create a new Macro frame)"
        n156 = call <vilib>:"Add State(s) to Queue__jki_lib_state_machine.vi"("State(s) in (\"\")"=w363) -> ("States Out"=w362:string)  [unwired: 14 in]
      }
      frame "Macro: Initialize" {
        w364 = "Data: Initialize\nInitialize Core Data\nUI: Initialize\nUI: Front Panel State >> Maximize\nCommunication: Open Serial\nCommunication: 读运行标志"  # Data: Initialize Initialize Core Data UI: Initialize UI: Front Panel State >> Maximize Communication: Open Serial Communication: 读运行标志
        # "Initialization Macro\n(This is called once, when the VI starts)"
        n157 = call <vilib>:"Add State(s) to Queue__jki_lib_state_machine.vi"("State(s) in Front (\"\")"=w364, "State(s) in (\"\")"=w368) -> ("States Out"=w367:string)  [unwired: 13 in]
      }
      frame "Macro: Exit" {
        # "Exit Macro\n(This is called once, when the VI exits)"
        n158 = Unbundle By Name(w375) -> ("Core.Close Panel on Exit?"=w374:bool)
        n159 = Select(t="UI: Front Panel State >> Close", s=w374, f="") -> (s? t:f=w371:string)
        n160 = call <vilib>:"Add State(s) to Queue__jki_lib_state_machine.vi"("State(s) in (\"\")"=w371, "State(s) at Back (\"\")"="Data: Cleanup\nExit") -> ("States Out"=w369:string)  [unwired: 13 in]
        n161 = call <vilib>:"Add State(s) to Queue__jki_lib_state_machine.vi"("State(s) in Front (\"\")"=w369, "State(s) in (\"\")"=w378) -> ("States Out"=w377:string)  [unwired: 13 in]
      }
      frame "---------- Communication ----------" {
        # "Template Separator\n(You can make a copy of, or modify, this frame)"
        n162 = call <vilib>:"Add State(s) to Queue__jki_lib_state_machine.vi"("State(s) in (\"\")"=w382) -> ("States Out"=w381:string)  [unwired: 14 in]
      }
      frame "Communication: Open Serial" {
        # "Your code here.\n(You can make a copy of, or modify, this frame)"
        n163 = call "读取配置文件.vi"("error in"=w391, "配置"="串口号") -> ("error out"=w390:errorcluster, "路径"=w389:string)  [unwired: 8 in]
        n164 = call "开机连接.vi"("error in"=w390, "波特率"=u32 19200, "串口号"=w389) -> ("error out"=w383:errorcluster, "连接成功"=w385:bool, "serial master instance"=w387:refnum<class "Modbus Master.lvclass">)  [unwired: 6 in]
        n165 = Bundle By Name(cluster=w388, "serial master instance"=w387, "连接成功"=w385) -> (w386:T7)
        n166 = call <vilib>:"Add State(s) to Queue__jki_lib_state_machine.vi"("State(s) in (\"\")"=w394) -> ("States Out"=w393:string)  [unwired: 14 in]
      }
      frame "Communication: 设备启动" {
        # "Your code here.\n(You can make a copy of, or modify, this frame)"
        n167 = Unbundle By Name(w400) -> ("serial master instance"=w401:refnum<class "Modbus Master.lvclass">, "连接成功"=w402:bool, "进站OK"=w395:bool)
        n168 = case shown="True" w395 {
          tunnel: w404 -> [w408 w418]
          tunnel: [w408 w417] -> w403
          tunnel: w402 -> [w409 w416]
          tunnel: w401 -> [_ w415]
          tunnel: [w409 w414] -> w399
          tunnel: FALSE ("正在运行") -> [w410 w413]
          tunnel: [w410 w412] -> w396
          tunnel: w395 -> [w407 _]
          frame False {
            n169 = case shown="False" w407 {
              frame False {
                n170 = One Button Dialog(message="产品未进站。" ("消息")) -> ()  [unwired: 1 in, 1 out]
              }
              frame True {
              }
            }
          }
          frame True {
            n171 = case shown="False" w413 {
              selector: w413 -> [_ w440]
              tunnel: w418 -> [w424 w441]
              tunnel: [w423 w441] -> w417
              tunnel: w416 -> [w422 w442]
              tunnel: w415 -> [w421 _]
              tunnel: [w420 w442] -> w414
              tunnel: [w419 w440] -> w412
              frame False {
                n172 = case shown="True" w422 {
                  tunnel: w424 -> [w425 w430]
                  tunnel: [w425 w429] -> w423
                  tunnel: w421 -> [_ w428]
                  tunnel: [_ w427] -> w420
                  tunnel: [_ TRUE] -> w419
                  frame False {
                  }
                  frame True {
                    n173 = stacked-sequence {
                      tunnel: w430 -> [_ w436 _ _]
                      tunnel: [_ w435 _ _] -> w429
                      tunnel: w428 -> [_ w434 _ _]
                      tunnel: [_ w433 _ _] -> w427
                      frame #0 {
                        n174 = local write "阻断通讯"(TRUE ("阻断通讯")) -> ()
                      }
                      frame #1 {
                        w432 = cluster{"地址":u16, "布尔":bool, "名称":string}[] [{"地址"=50, "布尔"=TRUE, "名称"="启动"}, {"地址"=51, "布尔"=FALSE, "名称"="停止"}]  # A写入线圈信息组
                        n175 = call "写入单个线圈.vi"("error in"=w436, "写入线圈信息组"=w432, "MB_实体"=w434) -> ("输出簇"=w435:errorcluster, "连接成功"=w433:bool)  [unwired: 7 in]
                      }
                      frame #2 {
                        n176 = local write "阻断通讯"(FALSE ("阻断通讯")) -> ()
                      }
                      frame #3 {
                        n177 = Format Date/Time String(time format string (%c)="%Y-%m-%d %H:%M:%S" ("EndTime")) -> (date/time string=w438:string)  [unwired: 2 in]
                        n178 = global write "Global.vi" "start_time"(w438) -> ()
                      }
                    }
                  }
                }
              }
              frame True {
              }
            }
          }
        }
        n179 = Bundle By Name(cluster=w400, "正在运行"=w396, "连接成功"=w399) -> (w398:T7)
        n180 = call <vilib>:"Add State(s) to Queue__jki_lib_state_machine.vi"("State(s) in (\"\")"=w406) -> ("States Out"=w405:string)  [unwired: 14 in]
      }
      frame "Communication: 设备停止" {
        # "Your code here.\n(You can make a copy of, or modify, this frame)"
        n181 = Unbundle By Name(w447) -> ("serial master instance"=w448:refnum<class "Modbus Master.lvclass">, "连接成功"=w449:bool)
        n182 = case shown="True" TRUE ("正在运行") {
          selector: TRUE ("正在运行") -> [w454 _]
          tunnel: w451 -> [w455 w462]
          tunnel: [w455 w461] -> w450
          tunnel: w449 -> [w456 w460]
          tunnel: w448 -> [_ w459]
          tunnel: [w456 w458] -> w446
          tunnel: [w454 w457] -> w444
          frame False {
          }
          frame True {
            n183 = case shown="True" w460 {
              tunnel: w462 -> [w464 w469]
              tunnel: [w464 w468] -> w461
              tunnel: w459 -> [_ w467]
              tunnel: [_ w466] -> w458
              tunnel: [FALSE FALSE] -> w457
              frame False {
              }
              frame True {
                n184 = stacked-sequence {
                  tunnel: w469 -> [_ w475 _]
                  tunnel: [_ w474 _] -> w468
                  tunnel: w467 -> [_ w473 _]
                  tunnel: [_ w472 _] -> w466
                  frame #0 {
                    n185 = local write "阻断通讯"(TRUE ("阻断通讯")) -> ()
                  }
                  frame #1 {
                    w471 = cluster{"地址":u16, "布尔":bool, "名称":string}[] [{"地址"=50, "布尔"=FALSE, "名称"="启动"}, {"地址"=51, "布尔"=TRUE, "名称"="停止"}]  # A写入线圈信息组
                    n186 = call "写入单个线圈.vi"("error in"=w475, "写入线圈信息组"=w471, "MB_实体"=w473) -> ("输出簇"=w474:errorcluster, "连接成功"=w472:bool)  [unwired: 7 in]
                  }
                  frame #2 {
                    n187 = local write "阻断通讯"(FALSE ("阻断通讯")) -> ()
                  }
                }
              }
            }
          }
        }
        n188 = Bundle By Name(cluster=w447, "正在运行"=w444, "连接成功"=w446) -> (w445:T7)
        n189 = call <vilib>:"Add State(s) to Queue__jki_lib_state_machine.vi"("State(s) in (\"\")"=w453) -> ("States Out"=w452:string)  [unwired: 14 in]
      }
      frame "Communication: 读运行标志" {
        n190 = Unbundle By Name(w478) -> ("serial master instance"=w477:refnum<class "Modbus Master.lvclass">)
        n191 = stacked-sequence {
          tunnel: w483 -> [_ w492 _]
          tunnel: [_ w491 _] -> w482
          tunnel: [_ w490 _] -> w481
          tunnel: [_ w489 _] -> w480
          tunnel: w477 -> [_ w487 _]
          frame #0 {
            n192 = local write "阻断通讯"(TRUE ("阻断通讯")) -> ()
          }
          frame #1 {
            w488 = T9 [{"地址"=507, "数量"=1, "名称"="1测试结束标志", "线圈组"=[]}]  # A读多组线圈信息组
            n193 = call "读线圈组.vi"("error in"=w492, "读多组线圈__输入"=w488, "MB_实体"=w487) -> ("输出簇"=w491:errorcluster, "正在运行"=w489:bool, "连接成功"=w490:bool)  [unwired: 6 in]
          }
          frame #2 {
            n194 = local write "阻断通讯"(FALSE ("阻断通讯")) -> ()
          }
        }
        n195 = Bundle By Name(cluster=w478, "连接成功"=w481, "正在运行"=w480) -> (w479:T7)
        n196 = call <vilib>:"Add State(s) to Queue__jki_lib_state_machine.vi"("State(s) in (\"\")"=w485) -> ("States Out"=w484:string)  [unwired: 14 in]
      }
      frame "---------- 设备状态采集 ----------" {
        # "Do not put any code in this frame.\n(it is a separator no-op)"
        n197 = call <vilib>:"Add State(s) to Queue__jki_lib_state_machine.vi"("State(s) in (\"\")"=w497) -> ("States Out"=w496:string)  [unwired: 14 in]
      }
      frame "通讯参数设置" {
        n198 = stacked-sequence {
          tunnel: w499 -> [_ w507 _]
          tunnel: [_ w504 _] -> w498
          frame #0 {
            n199 = local write "阻断通讯"(TRUE ("阻断通讯")) -> ()
          }
          frame #1 {
            n200 = call "通讯参数设置.vi"() -> ("A设备簇"=w508:T8)  [unwired: 5 in]
            n201 = Unbundle By Name(w508) -> ("MB_实体"=w506:refnum<class "Modbus Master.lvclass">, "连接成功"=w505:bool)
            n202 = Bundle By Name(cluster=w507, "serial master instance"=w506, "连接成功"=w505) -> (w504:T7)
          }
          frame #2 {
            n203 = local write "阻断通讯"(FALSE ("阻断通讯")) -> ()
          }
        }
        n204 = call <vilib>:"Add State(s) to Queue__jki_lib_state_machine.vi"("State(s) in (\"\")"=w502) -> ("States Out"=w501:string)  [unwired: 14 in]
      }
    }
  }
  n205 = while {
    tunnel: w1 -> [w513]
    stop <- w510 stop-if-true
    n206 = call "Read From Console.vi"("error in (no error)"=w513) -> ("Output"=→"消息框+":string)  [unwired: 9 in, 1 out]
    n207 = property on="消息框+" class="Str"("Text.Scroll Position"=i8 -1 ("milliseconds to wait")) -> ()  [unwired: 2 in, 2 out]
    n208 = Wait (ms)(milliseconds to wait=u32 20 ("等待时间（毫秒）")) -> ()  [unwired: 1 out]
    n209 = local read "Exit"() -> (w510:bool)
  }
